vi "Read Offset.vi"(8 "error in (no error)":errorcluster, 11 "MatchPattern_STR in":refnum<class "MatchPattern_STR.lvclass">) -> (0 "error out":errorcluster, 2 "Offset":i32, 3 "MatchPattern_STR out":refnum<class "MatchPattern_STR.lvclass">)   [LabVIEW 2021, in "MatchPattern_STR.lvclass"]
uses:
  MatchPattern_STR.lvclass
  MatchPattern_STR.lvclass/MatchPattern_STR.ctl
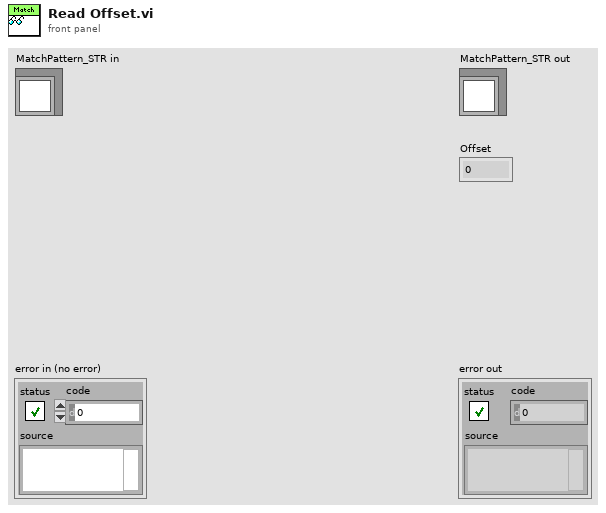
[diagram p1: front panel]
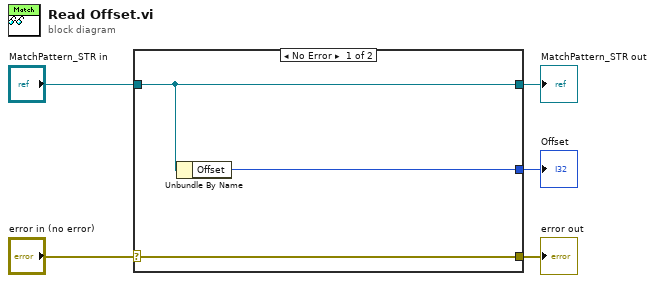
[diagram p0: block diagram]
diagram:
  n1 = case shown="No Error" "error in (no error)" {
    selector: "error in (no error)" -> [w8 w9]
    tunnel: [w8 w9] -> w4
    tunnel: [w7 w10] -> w2
    tunnel: "MatchPattern_STR in" -> [w7 w10]
    tunnel: [w6 _] -> w1
    frame No Error {
      n2 = Unbundle By Name(w7) -> ("Offset"=w6:i32)
    }
    frame Error {
    }
  }
  "error out" <- w4
  "MatchPattern_STR out" <- w2
  "Offset" <- w1
